vi "Output DMA Engine.vi"(10 "Parameters":variant, 11 "Process":refnum<class "Process.lvclass">) -> ()   [LabVIEW 2016, in "FPGA Addon Engine.lvlib"]
uses:
  FPGA Addon Engine.lvlib
  <vilib>/NI/NIVS Inline Async API/_VS Inline Async API/Process/Process.lvclass
  Types/DMA Output References.ctl
  <vilib>/NI Veristand/Custom Device Waveform API/Single Waveform Read (DBL)/Single Waveform Read (DBL).lvclass
  Types/DMA Output Ref.ctl
  <vilib>/NI/NIVS Inline Async API/_VS Inline Async API/Process/Process.lvclass/Process.ctl
  <vilib>/Platform/TimedLoop/XDataNode/timing_clust.ctl
  <vilib>/Platform/TimedLoop/XDataNode/nitl_modes.ctl
  <vilib>/Platform/TimedLoop/XDataNode/wakeup.ctl
  <vilib>/NI/NIVS Inline Async API/_Data Access Engine/Access Type Classes/Write/Write.lvclass/Write.ctl
  <vilib>/NI/NIVS Inline Async API/_Data Access Engine/Data Access Engine/Methods/Write.Data.vi
  <vilib>/NI/NIVS Inline Async API/_VS Inline Async API/Process/Data Member Access/Read Data Access.vi
  <vilib>/NI/NIVS Inline Async API/_VS Inline Async API/Error Handling Process/SubVIs/Error.ConvertArray.vi
  <vilib>/NI/NIVS Inline Async API/_Data Access Engine/Access Type Classes/Write/Write.ProcessData.vi
  <vilib>/NI Veristand/Custom Device Waveform API/Single Waveform Read (DBL)/NI VeriStand - Close Single Waveform Read Session (DBL).vi
  <vilib>/FPGAPlugInAG/Dynamic/niLvFpga_Close_Dynamic.vi
  <vilib>/NI/NIVS Inline Async API/_Data Access Engine/Data Access Engine/Methods/Write.Lookup.vi
  <vilib>/rvi/interface/nirviCloseFPGA/nirviCloseFPGA.xnode
  <vilib>/Platform/TimedLoop/XDataNode/XDataNode.xnode
  <vilib>/NI/NIVS Inline Async API/_Data Access Engine/Data Access Engine/Data Access Engine.lvclass
  <vilib>/NI VeriStand/Custom Device Waveform API/NI_VS Custom Device Waveform API.lvlib
  <vilib>/NI VeriStand/Custom Device Tools/Custom Device Utility Library/Custom Device Utility Library.lvlib
  <vilib>/Platform/TimedLoop/XDataNode/XDNodeRunTimeDep.lvlib
panel:
  out "error out":errorcluster
  in  "error in (no error)":errorcluster
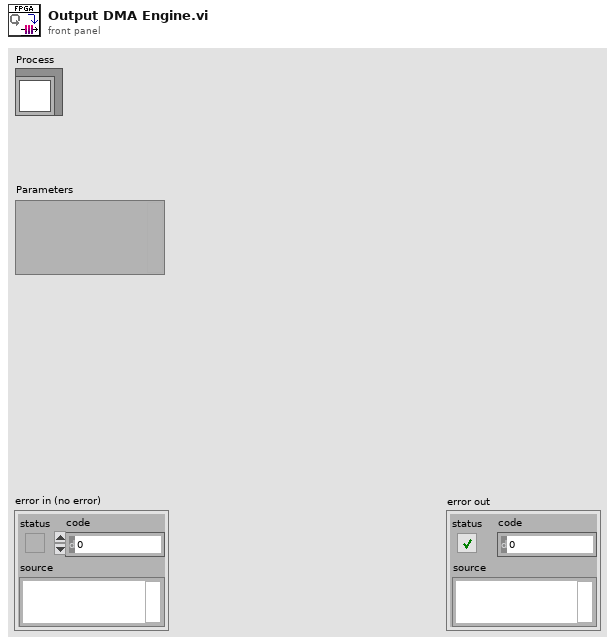
[diagram p1: front panel]
types:
  T1 = typedef "FPGA Addon Engine.lvlib/DMA Output References.ctl" = cluster{"Waveforms":refnum<class "Single Waveform Read (DBL).lvclass">[], "DMA Ref":T2, "Name":string}
  T2 = typedef "FPGA Addon Engine.lvlib/DMA Output Ref.ctl" = refnum<k20>
  T3 = typedef "Data Access Engine.lvlib/Data Access Engine.lvclass/Write.DVR.ctl" = refnum<data-value>
  T4 = typedef "XDNodeRunTimeDep.lvlib/timing_clust.ctl" = cluster{"Expected End [f-1]":u64, "Actual End [f-1]":u64, "Finished Late? [f-1]":bool, "Expected End [i-1]":u64, "Actual End [i-1]":u64, "Finished Late? [i-1]":bool, "Expected Start [i]":u64, "Actual Start [i]":u64, "Expected Start [f]":u64, "Actual Start [f]":u64, "Source Name":string, "Structure Name":string, "Period":i64, "Deadline":i64, "Offset":i64, "Start":i64, "Priority":i32, "Timeout":i32, "Mode":T5, "Wakeup Reason":T6, "Error":errorcluster, "Source Type":string, "Secondary Source Type":string, "Global End Time":u64, "Global Start Time":u64, "Frame Duration":u64, "Iteration Duration":u64, "Assigned CPU":i32, "I/O Scan Engine Mode":u32}
  T5 = typedef "XDNodeRunTimeDep.lvlib/nitl_modes.ctl" = enum32{"No Change", "Process missed periods, maintain original phase", "Discard missed periods, maintain original phase", "Process missed periods, ignore original phase", "Discard missed periods, ignore original phase"}
  T6 = typedef "XDNodeRunTimeDep.lvlib/wakeup.ctl" = enum32{"Normal", "Aborted", "Asynchronous wakeup", "Timing source error", "Timed loop error", "Timeout"}
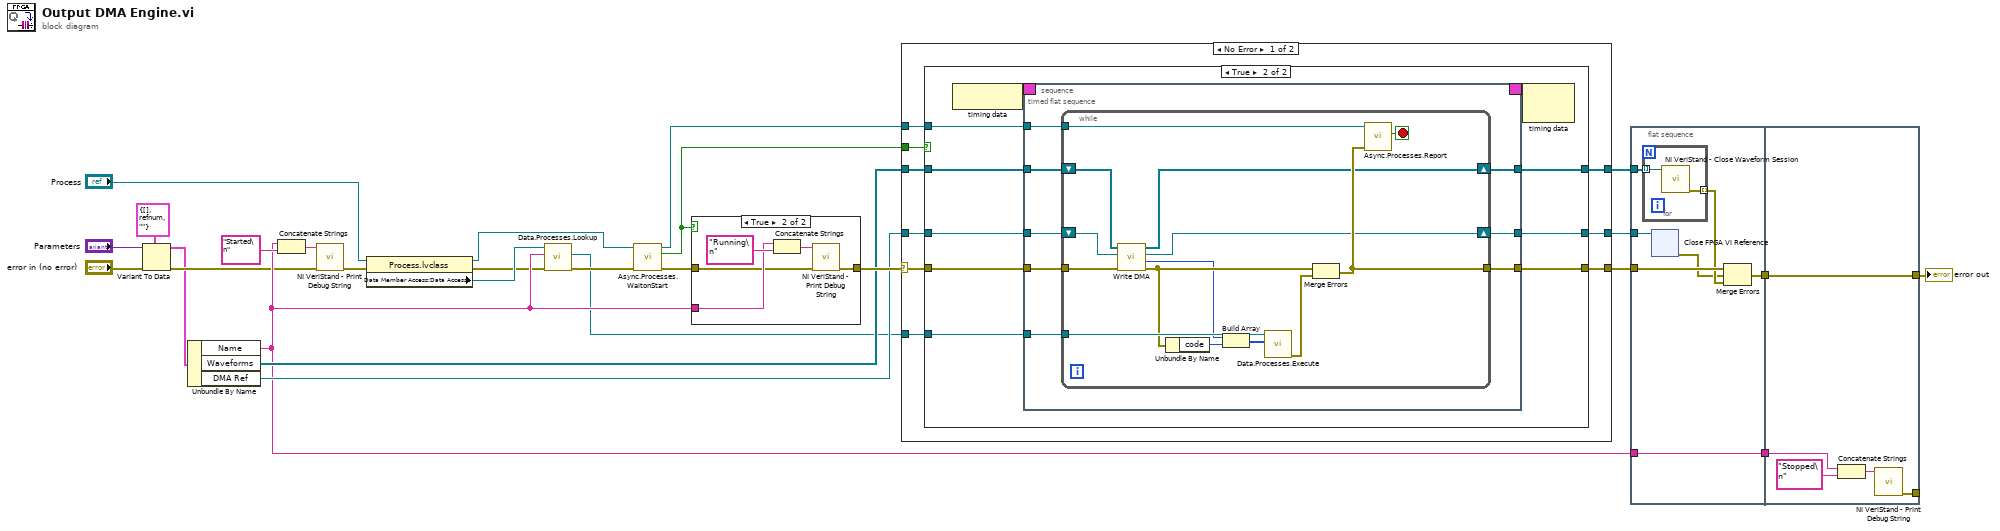
[diagram p0: block diagram]
diagram:
  n1 = Variant To Data(error in="error in (no error)", type=T1 {"Waveforms"=[], "DMA Ref"=refnum, "Name"=""} ("Parameters"), Variant="Parameters") -> (data=w2:T1, error out=w4:errorcluster)
  n2 = Unbundle By Name(w2) -> ("Name"=w9:string, "Waveforms"=w17:refnum<class "Single Waveform Read (DBL).lvclass">[], "DMA Ref"=w16:T2)
  n3 = Concatenate Strings(w9, "Started\n" ("string")) -> (w23:string)
  n4 = call <vilib>:"NI VeriStand - Print Debug String.vi"("error in (no error)"=w4, "Message"=w23) -> ("error out"=w10:errorcluster)  [unwired: 9 in]
  n5 = property class="Process.lvclass"(reference="Process", error in=w10) -> (reference out=w11:refnum<class "Process.lvclass">, error out=w7:errorcluster, "Data Member Access:Data Access"=w8:refnum<class "Data Access Engine.lvclass">)
  n6 = call-poly <vilib>:"Data.Processes.Lookup.vi"("error in (no error)"=w7, "Name"=w9, "Data Access API in"=w8) -> ("error out"=w6:errorcluster, "Ref"=w5:T3)  [unwired: 5 in, 2 out]
  n7 = call <vilib>:"Async.Processes.WaitonStart.vi"("error in (no error)"=w6, "Process"=w11) -> ("error out"=w14:errorcluster, "Execute"=w15:bool, "Process out"=w13:refnum<class "Process.lvclass">)  [unwired: 7 in]
  n8 = case shown="True" w15 {
    tunnel: w9 -> [_ w31]
    tunnel: w14 -> [w28 w30]
    tunnel: [w28 w29] -> w20
    frame False {
    }
    frame True {
      n9 = Concatenate Strings(w31, "Running\n" ("string")) -> (w33:string)
      n10 = call <vilib>:"NI VeriStand - Print Debug String.vi"("error in (no error)"=w30, "Message"=w33) -> ("error out"=w29:errorcluster)  [unwired: 9 in]
    }
  }
  n11 = case shown="No Error" w20 {
    selector: w20 -> [w39 w90]
    tunnel: [w42 w92] -> w25
    tunnel: [w41 w90] -> w24
    tunnel: w13 -> [w40 _]
    tunnel: w15 -> [w38 _]
    tunnel: [w37 w91] -> w21
    tunnel: w5 -> [w36 _]
    tunnel: w17 -> [w35 w92]
    tunnel: w16 -> [w34 w91]
    frame No Error {
      n12 = case shown="True" w38 {
        tunnel: [w43 w55] -> w42
        tunnel: [w45 w54] -> w41
        tunnel: w40 -> [_ w53]
        tunnel: w39 -> [w45 w52]
        tunnel: [w44 w51] -> w37
        tunnel: w36 -> [_ w50]
        tunnel: w35 -> [w43 w49]
        tunnel: w34 -> [w44 w48]
        frame False {
        }
        frame True {
          n13 = node-c288() -> (w47:T4)
          n14 = timed-sequence {
            timing: w47 -> [_]
            timing-out: [_] -> w46
            tunnel: [w63] -> w55
            tunnel: [w62] -> w54
            tunnel: w53 -> [w61]
            tunnel: w52 -> [w60]
            tunnel: [w59] -> w51
            tunnel: w50 -> [w58]
            tunnel: w49 -> [w57]
            tunnel: w48 -> [w56]
            n15 = timed-flat-sequence {
              tunnel: [w71] -> w63
              tunnel: [w70] -> w62
              tunnel: w61 -> [w69]
              tunnel: w60 -> [w68]
              tunnel: [w67] -> w59
              tunnel: w58 -> [w66]
              tunnel: w57 -> [w65]
              tunnel: w56 -> [w64]
              n16 = while {
                tunnel: w69 -> [w85]
                tunnel: w66 -> [w82]
                shift-right: [w73] -> w67
                shift-left: w64 -> [w75]
                shift-right: [w79] -> w71
                shift-left: w65 -> [w76]
                tunnel: w68 -> [w78]
                tunnel: [w80] -> w70
                stop <- w72 stop-if-true
                n17 = call "Write DMA.vi"("error in (no error)"=w78, "DMA Ref"=w75, "Waveform Refs"=w76) -> ("error out"=w77:errorcluster, "Empty Elements Remaining"=w74:u32, "DMA Ref"=w73:T2, "Waveform Refs"=w79:refnum<class "Single Waveform Read (DBL).lvclass">[])  [unwired: 5 in]
                n18 = Unbundle By Name(w77) -> ("code"=w84:i32)
                n19 = Build Array(w74, w84) -> (w83:u32[])
                n20 = call-poly <vilib>:"Data.Processes.Execute.vi"("Values"=w83, "Ref"=w82) -> ("error out"=w81:errorcluster)  [unwired: 9 in]
                n21 = Merge Errors(w77, w81) -> (w80:errorcluster)
                n22 = call <vilib>:"Async.Processes.Report.vi"("Error"=w80, "Process in"=w85) -> ("Stop"=w72:bool)  [unwired: 8 in, 1 out]
              }
            }
          }
          n23 = node-c288(w46) -> ()  [unwired: 1 out]
        }
      }
    }
    frame Error {
    }
  }
  n24 = flat-sequence {
    tunnel: w25 -> [w99]
    tunnel: w24 -> [w98]
    tunnel: w21 -> [w95]
    tunnel: [w96] -> w27
    tunnel: [w93] -> w26
    tunnel: w9 -> [w93]
    tunnel: [w106] -> w18
    tunnel: w27 -> [w106]
    tunnel: w26 -> [w103]
    tunnel: [w102] -> _
    frame #0 {
      n25 = for {
        tunnel: w99 -> [w101] mode=indexing
        tunnel: [w100] -> w97 mode=indexing
        n26 = call-poly <vilib>:"NI VeriStand - Close Waveform Session.vi"("Single Waveform Read Session (DBL)"=w101) -> ("error out"=w100:errorcluster)  [unwired: 10 in]
      }
      n27 = xnode "Close FPGA VI Reference"("FPGA VI Reference In"=w95) -> ("error out"=w94:errorcluster)  [unwired: 1 in]
      n28 = Merge Errors(w98, w94, w97) -> (w96:errorcluster)
    }
    frame #1 {
      n29 = Concatenate Strings(w103, "Stopped\n" ("string")) -> (w104:string)
      n30 = call <vilib>:"NI VeriStand - Print Debug String.vi"("Message"=w104) -> ("error out"=w102:errorcluster)  [unwired: 10 in]
    }
  }
  "error out" <- w18
